vi "Read Message Tag.vi"(8 "error in (no error)":errorcluster, 11 "abs_EventLog in":refnum<class "abs_EventLog.lvclass">) -> (0 "error out":errorcluster, 2 "Message Tag":string, 3 "abs_EventLog out":refnum<class "abs_EventLog.lvclass">)   [LabVIEW 2021, in "abs_EventLog.lvclass"]
uses:
  abs_EventLog.lvclass
  abs_EventLog.lvclass/abs_EventLog.ctl
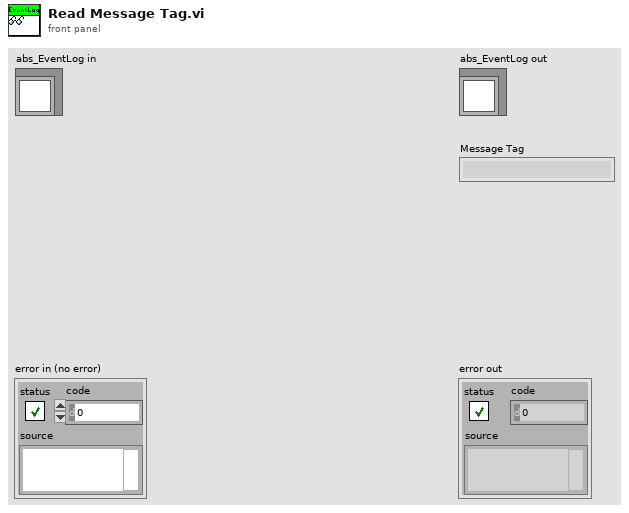
[diagram p1: front panel]
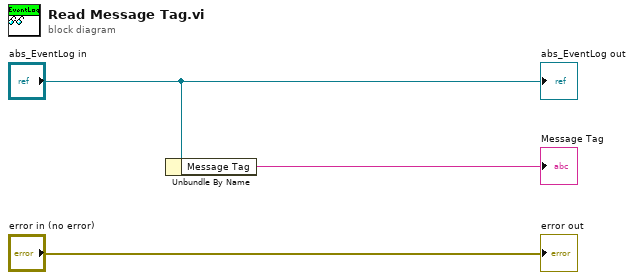
[diagram p0: block diagram]
diagram:
  n1 = Unbundle By Name("abs_EventLog in") -> ("Message Tag"=→"Message Tag":string)
  "error out" <- "error in (no error)"
  "abs_EventLog out" <- "abs_EventLog in"
